vi "readImageNumber.vi"(8 "error in (no error)":errorcluster, 10 "NativeXML in":refnum<class "NativeXML.lvclass">, 11 "WinX32Settings in":refnum<class "WinX32Settings.lvclass">) -> (0 "error out":errorcluster, 2 "NativeXML out":refnum<class "NativeXML.lvclass">, 3 "WinX32Settings out":refnum<class "WinX32Settings.lvclass">)   [LabVIEW 2011, in "Tools.lvlib" / "Settings.lvlib" / "WinX32Settings.lvclass"]
uses:
  WinX32Settings.lvclass
  NativeXML/NativeXML.lvclass
  WinX32Settings.lvclass/WinX32Settings.ctl
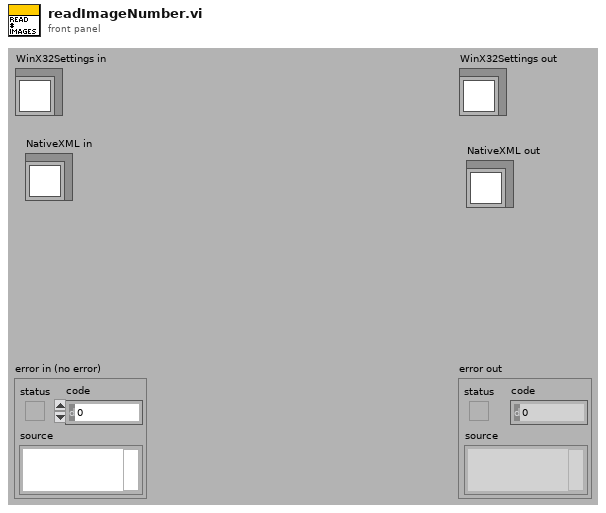
[diagram p1: front panel]
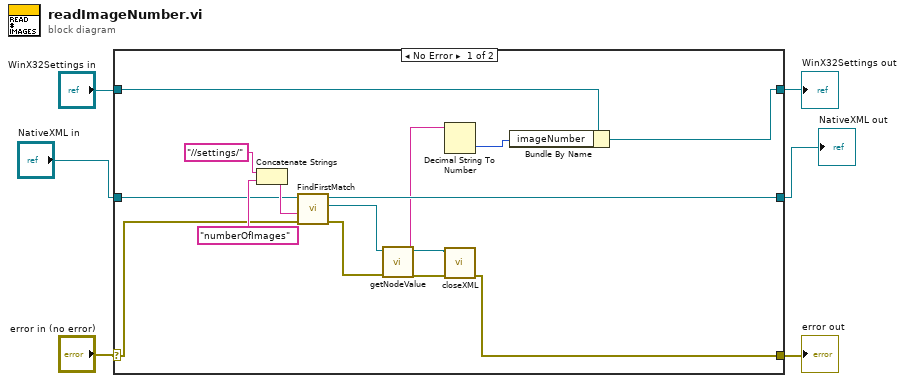
[diagram p0: block diagram]
diagram:
  n1 = case shown="No Error" "error in (no error)" {
    selector: "error in (no error)" -> [w11 w22]
    tunnel: [w17 w22] -> w1
    tunnel: [w20 w23] -> w5
    tunnel: "WinX32Settings in" -> [w21 w23]
    tunnel: "NativeXML in" -> [w9 w24]
    tunnel: [w14 w24] -> w4
    frame No Error {
      n2 = Concatenate Strings("//settings/" ("searchElementIn"), "numberOfImages") -> (w10:string)
      n3 = call "FindFirstMatch.vi"("error in (no error)"=w11, "xPath"=w10, "NativeXML in"=w9) -> ("error out"=w12:errorcluster, "NativeXML match"=w13:refnum<class "NativeXML.lvclass">, "NativeXML out"=w14:refnum<class "NativeXML.lvclass">)  [unwired: 6 in]
      n4 = call "getNodeValue.vi"("error in (no error)"=w12, "NativeXML in"=w13) -> ("error out"=w18:errorcluster, "Value"=w7:string, "NativeXML out"=w19:refnum<class "NativeXML.lvclass">)  [unwired: 7 in]
      n5 = Decimal String To Number(string=w7) -> (number=w8:i32)  [unwired: 2 in, 1 out]
      n6 = call "closeXML.vi"("error in (no error)"=w18, "NativeXML in"=w19) -> ("error out"=w17:errorcluster)  [unwired: 9 in]
      n7 = Bundle By Name(cluster=w21, "imageNumber"=w8) -> (w20:refnum<class "WinX32Settings.lvclass">)
    }
    frame Error {
    }
  }
  "error out" <- w1
  "WinX32Settings out" <- w5
  "NativeXML out" <- w4
